vi "Pin Positions 2 Selected.vi"(10 "Pin":T1[](array[typedef])) -> (2 "Selected":T2[](array[typedef]))   [LabVIEW 2013]
uses:
  Selected Pin Positions.ctl
  lib/Data Access Objects/Metadata/Pin Positions.ctl
panel:
  # "Fixed"
  # "Platten"
  # "X"
  # "Z"
  # "X"
  # "Z"
  # "Y"
  # "Y"
  # "Fixed"
  # "Platten"
  # "X"
  # "Z"
  # "X"
  # "Z"
  # "Y"
  # "Y"
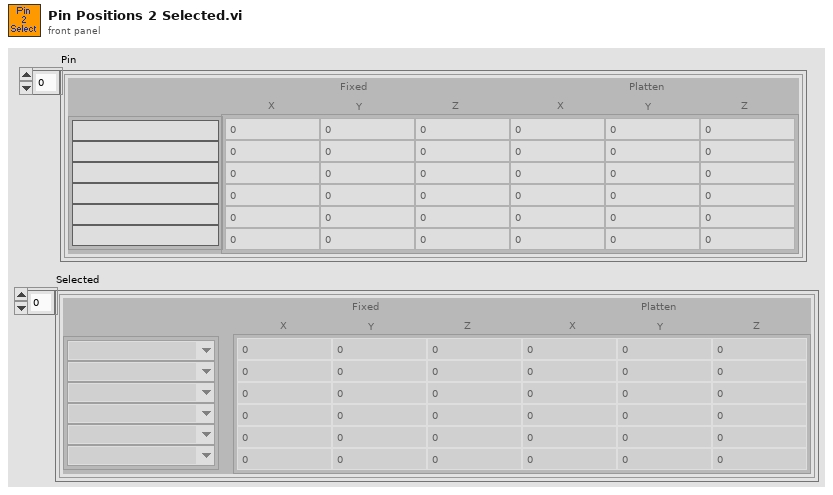
[diagram p1: front panel]
types:
  T1 = typedef "Pin Positions.ctl" = cluster{"Pin Positions":dbl[][], "Row Labels":string[]}
  T2 = typedef "Selected Pin Positions.ctl" = cluster{"Pin Positions":dbl[][], "Row Labels":u16[]}
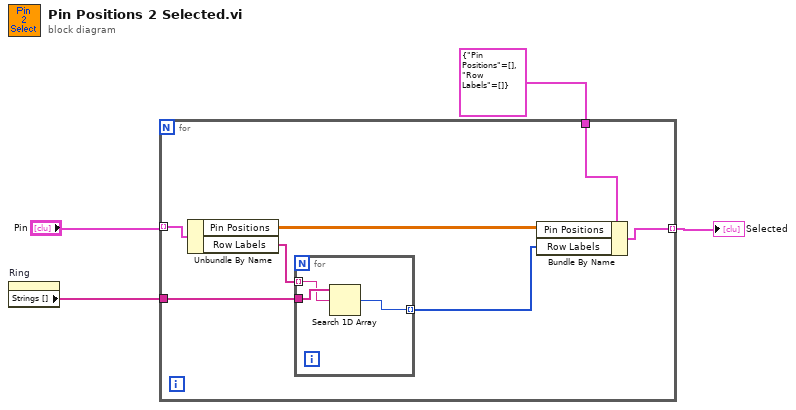
[diagram p0: block diagram]
diagram:
  n1 = property on="Ring" class="Ring (strict)"() -> ("Strings []"=w4:string[])  [unwired: 2 in, 2 out]
  n2 = for {
    tunnel: "Pin" -> [w11] mode=indexing
    tunnel: w4 -> [w10]
    tunnel: T2 {"Pin Positions"=[], "Row Labels"=[]} ("PinPositions") -> [w8]
    tunnel: [w5] -> w1 mode=indexing
    n3 = Unbundle By Name(w11) -> ("Pin Positions"=w7:dbl[][], "Row Labels"=w9:string[])
    n4 = for {
      tunnel: w10 -> [w13]
      tunnel: w9 -> [w12] mode=indexing
      tunnel: [w14] -> w6 mode=indexing
      n5 = Search 1D Array(1D array=w13, element=w12) -> (index of element=w14:i32)  [unwired: 1 in]
    }
    n6 = Bundle By Name(cluster=w8, "Pin Positions"=w7, "Row Labels"=w6) -> (w5:T2)
  }
  "Selected" <- w1
